vi "test2.vi"() -> ()   [LabVIEW 2014]
panel:
  in  "?":bool
  out "v":dbl
  in  "h":dbl
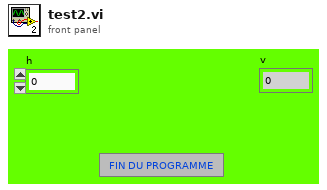
[diagram p1: front panel]
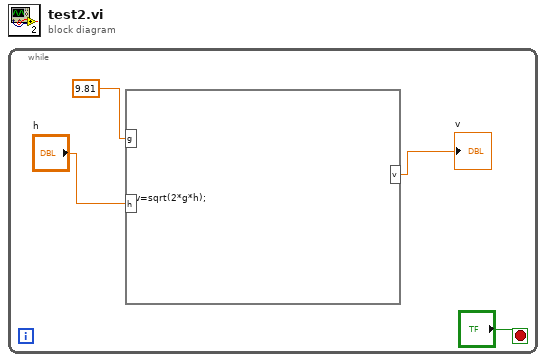
[diagram p0: block diagram]
diagram:
  n1 = while {
    stop <- "?" stop-if-true
    n2 = formula code="v=sqrt(2*g*h);"("g"=9.81, "h"="h") -> ("v"=→"v":dbl)
  }
